vi "SWITCH Digital Path Generation Cases Individual.vi"() -> ()   [LabVIEW 2021]
uses:
  <instrlib>/niSwitch/niSwitch.llb/niSwitch Topologies.ctl
  Static Digital Path Generation/Typedefs/Module Characteristics.ctl
  Static Digital Path Generation/Typedefs/Terminal and State Settings.ctl
  Static Digital Path Generation/Typedefs/Path Status.ctl
  Static Digital Path Generation/Switch_Static Digital Path Generation.lvlib
panel:
  out "Path Status 1":T1=3 items=["Other", "Path Available", "Path Exists", "Path Unsupported", "Resource in Use", "Source Conflict", "Channel Not Available"]
  in  "Terminal and State Settings 1":T2={"Connect/Disconnect"=TRUE, "Channel 1"="ch0", "Channel 2"="ch1"}
  out "error out":errorcluster
  out "Path Status 2":T1=1 items=["Other", "Path Available", "Path Exists", "Path Unsupported", "Resource in Use", "Source Conflict", "Channel Not Available"]
  in  "Terminal and State Settings 2":T2={"Connect/Disconnect"=TRUE, "Channel 1"="ch0", "Channel 2"="com0"}
  out "Path Status 3":T1=4 items=["Other", "Path Available", "Path Exists", "Path Unsupported", "Resource in Use", "Source Conflict", "Channel Not Available"]
  in  "Terminal and State Settings 3":T2={"Connect/Disconnect"=TRUE, "Channel 1"="ch1", "Channel 2"="com0"}
  out "Module Characteristics":T3={" Max. DC Voltage (V)"=300.0, "Max. Switching DC Current (A)"=2.0, "Max. AC Voltage (V)"=300.0, "Max. Switching AC Current (A)"=2.0}
  in  "Topology Name":T4="2527/2-Wire Dual 16x1 Mux"
  in  "Switch Resource Name":refnum<k15>="MUX_2527"
  # "* Works with Matrix Topology"
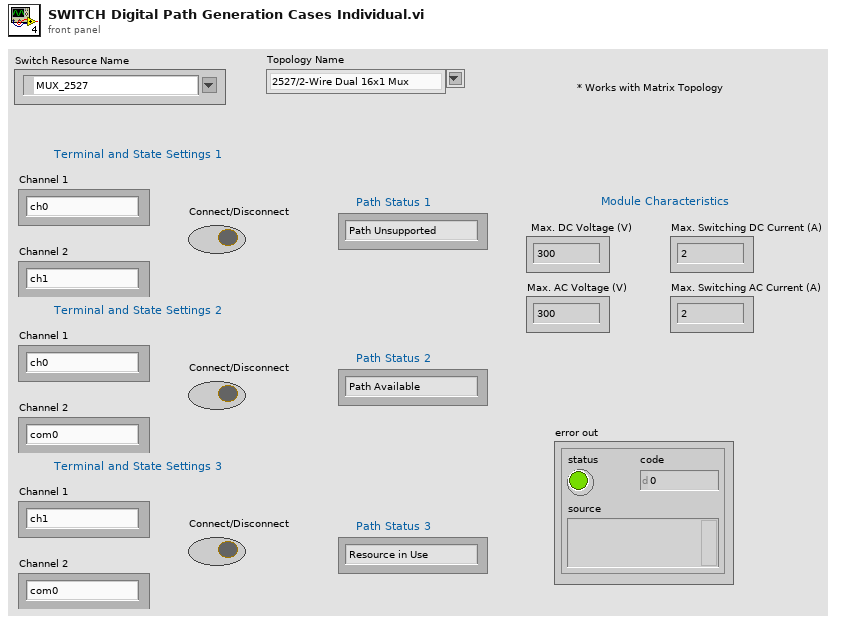
[diagram p1: front panel]
types:
  T1 = typedef "Switch_Static Digital Path Generation.lvlib/Path Status.ctl" = i32
  T2 = typedef "Switch_Static Digital Path Generation.lvlib/Terminal and State Settings.ctl" = cluster{"Connect/Disconnect":bool, "Channel 1":string, "Channel 2":string}
  T3 = typedef "Switch_Static Digital Path Generation.lvlib/Module Characteristics.ctl" = cluster{" Max. DC Voltage (V)":dbl, "Max. Switching DC Current (A)":dbl, "Max. AC Voltage (V)":dbl, "Max. Switching AC Current (A)":dbl}
  T4 = typedef "niSwitch Topologies.ctl" = string
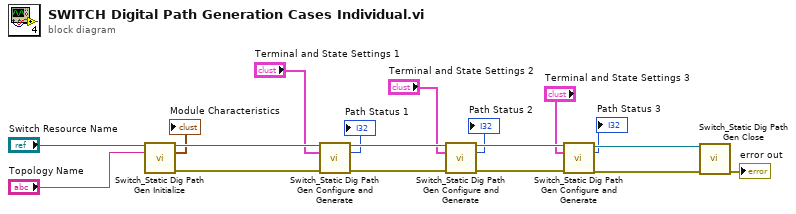
[diagram p0: block diagram]
diagram:
  n1 = call "Switch_Static Dig Path Gen Initialize.vi"("Switch Resource Name"="Switch Resource Name", "Topology Name"="Topology Name") -> ("Switch Handle Out"=w18:refnum<k15>, "Module Characteristics"=→"Module Characteristics":T3, "error out"=w17:errorcluster)  [unwired: 11 in]
  n2 = call "Switch_Static Dig Path Gen Configure and Generate.vi"("Switch Handle In"=w18, "Terminal and State Settings"="Terminal and State Settings 1", "error in"=w17) -> ("Switch Handle Out"=w16:refnum<k15>, "Path Status"=→"Path Status 1":T1, "error out"=w15:errorcluster)  [unwired: 10 in]
  n3 = call "Switch_Static Dig Path Gen Configure and Generate.vi"("Switch Handle In"=w16, "Terminal and State Settings"="Terminal and State Settings 2", "error in"=w15) -> ("Switch Handle Out"=w14:refnum<k15>, "Path Status"=→"Path Status 2":T1, "error out"=w13:errorcluster)  [unwired: 10 in]
  n4 = call "Switch_Static Dig Path Gen Configure and Generate.vi"("Switch Handle In"=w14, "Terminal and State Settings"="Terminal and State Settings 3", "error in"=w13) -> ("Switch Handle Out"=w12:refnum<k15>, "Path Status"=→"Path Status 3":T1, "error out"=w11:errorcluster)  [unwired: 10 in]
  n5 = call "Switch_Static Dig Path Gen Close.vi"("Switch Handle In"=w12, "error in"=w11) -> ("error out"=→"error out":errorcluster)  [unwired: 13 in]
